vi "Abort Channel.vi"(8 "sync in":errorcluster) -> (3 "Channel out":T1)   [LabVIEW 2025]
uses:
  <extravilib>/ChannelInstances/Event Messenger-c(str,var)/))Channel.ctl
  <extravilib>/ChannelInstances/Event Messenger-c(str,var)/))Channel.vi
  <extravilib>/ChannelInstances/Event Messenger-c(str,var).lvlib
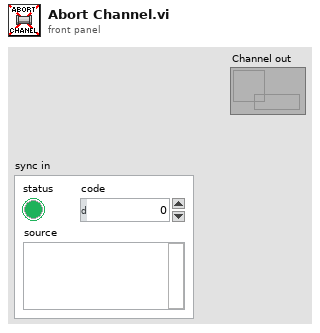
[diagram p1: front panel]
types:
  T1 = typedef "Event Messenger-c(str,var).lvlib/))Channel.ctl" = refnum<queue>
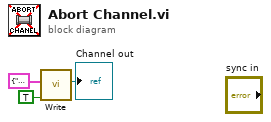
[diagram p0: block diagram]
diagram:
  n1 = call <extravilib>:"Write.vi"("abort (F)"=TRUE, "element"=cluster{"cmd":string, "data":variant} {"cmd"="", "data"=variant}) -> ("channel"=→"Channel out":T1)  [unwired: 8 in, 1 out]
